vi "Load 16bit Image Stack from Tiff.vi"(0 "path to TIFF file":path=path "/HD1/Users/herbertlooser/Desktop/Ladungsspr焗er.tif", 1 "error in (no error)":errorcluster) -> (5 "I16":i16[][][](array[numeric]), 6 "Directories":cluster{"Tags":T1[]}[](array[cluster]), 7 "error out":errorcluster)   [LabVIEW 2015, in "Tiff reader.lvlib"]
doc: "This .vi is taken from an online tiff reader. It is able to read I16-bit .tiff images."
uses:
  Tiff reader.lvlib
  FieldTypes.ctl
  IFD Entry.ctl
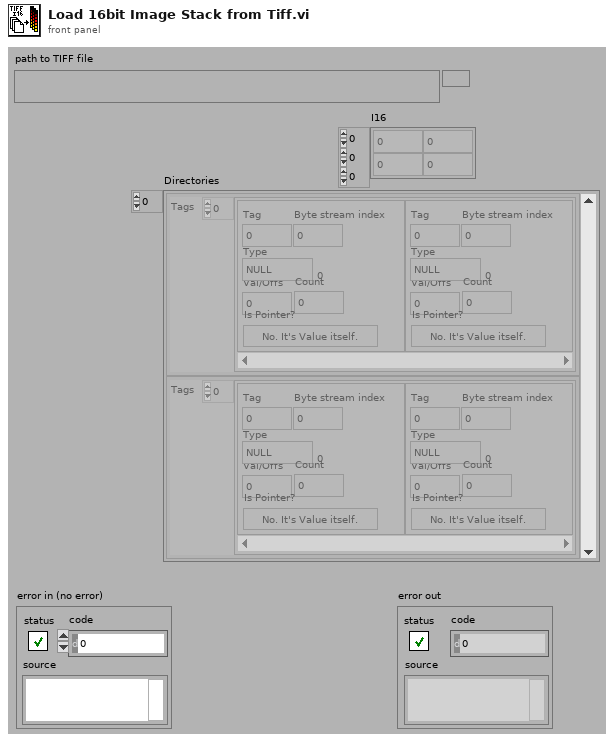
[diagram p1: front panel]
types:
  T1 = typedef "Tiff reader.lvlib/IFD Entry.ctl" = cluster{"Tag":u16, "Type":T2, "Count":u32, "Val/Offs":u32, "Is Pointer?":bool, "Byte stream index":i32}
  T2 = typedef "Tiff reader.lvlib/FieldTypes.ctl" = enum16{"NULL", "U8", "ASCII7", "U16", "U32", "RATIONAL", "SByte(I8)", "Undef(8Bit)", "I16", "I32", "SRat(4B:4B)", "SGL(4Byte)", "DBL(8Byte)"}
  T3 = enum16{"open", "open or create", "create or replace", "create"}
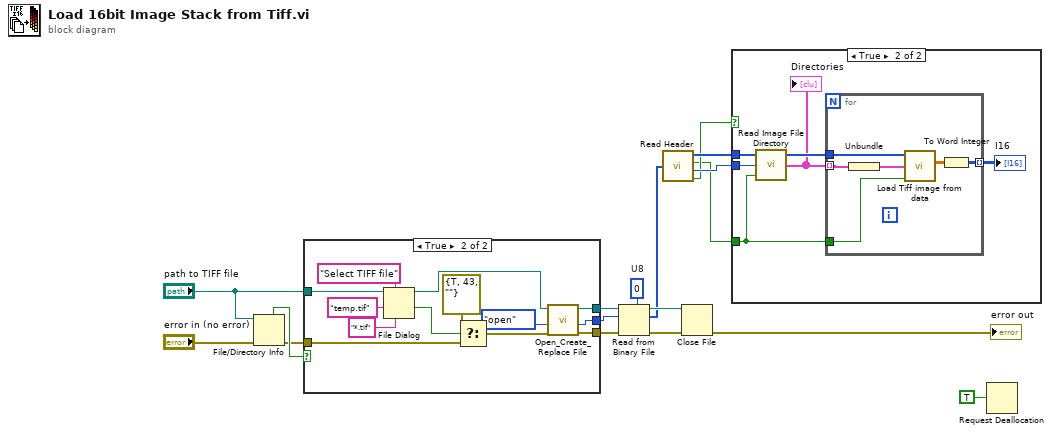
[diagram p0: block diagram]
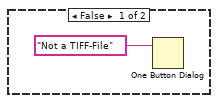
[diagram p2: hidden frame]
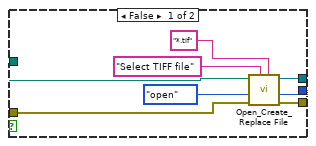
[diagram p3: hidden frame]
diagram:
  w1 = u8 0  # U8
  n1 = File/Directory Info(path="path to TIFF file", error in="error in (no error)") -> (directory=w12:bool, error out=w4:errorcluster)  [unwired: 5 out]
  n2 = case shown="True" w12 {
    tunnel: [w22 w31] -> w17
    tunnel: [w21 w33] -> w16
    tunnel: [w20 w32] -> w13
    tunnel: w4 -> [w19 w29]
    tunnel: "path to TIFF file" -> [w18 w27]
    frame False {
      n3 = call <vilib>:"Open_Create_Replace File.vi"("pattern"="*.tif", "prompt"="Select TIFF file", "error in (no error)"=w19, "function (open:0)"=T3."open", "file path"=w18) -> ("error out"=w20:errorcluster, "file size (bytes)"=w22:i32, "refnum"=w21:refnum<file>)  [unwired: 2 in, 2 out]
    }
    frame True {
      n4 = File Dialog(6:"*.tif" ("pattern"), 7:"Select TIFF file" ("prompt"), 9:"temp.tif" ("default name"), 11:w27) -> (1:w30:bool, 3:w35:path)  [unwired: 1 in, 4 out]
      n5 = Select(t=errorcluster {"status"=TRUE, "code"=43, "source"=""} ("error in (no error)"), s=w30, f=w29) -> (s? t:f=w28:errorcluster)
      n6 = call <vilib>:"Open_Create_Replace File.vi"("error in (no error)"=w28, "function (open:0)"=T3."open", "file path"=w35) -> ("error out"=w32:errorcluster, "file size (bytes)"=w31:i32, "refnum"=w33:refnum<file>)  [unwired: 3 in, 3 out]
    }
  }
  n7 = Read from Binary File(5:w1, 8:w13, 10:w17, 11:w16) -> (0:w14:errorcluster, 2:w2:u8[], 3:w15:refnum<file>)  [unwired: 3 out]
  n8 = call "Read Header.vi"("TIFF Data in"=w2) -> ("TIFF Data out"=w10:u8[], "Litt/BigEnd"=w7:bool, "ImFileDirectOffs"=w9:u32, "IsTIFF?"=w8:bool)
  n9 = Close File(refnum=w15, error in=w14) -> (error out=→"error out":errorcluster)  [unwired: 1 out]
  n10 = case shown="True" w8 {
    tunnel: w10 -> [_ w45]
    tunnel: w9 -> [_ w44]
    tunnel: w7 -> [_ w42]
    frame False {
      n11 = One Button Dialog(message="Not a TIFF-File") -> ()  [unwired: 2 out]
    }
    frame True {
      n12 = call "Read Image File Directory.vi"("Litt/BigEnd"=w42, "Im_File_Dir Offs"=w44, "Image Data in"=w45) -> ("Directories"=w40:cluster{"Tags":T1[]}[], "Image Data out"=w43:u8[])  [unwired: 1 out]
      "Directories" <- w40
      n13 = for {
        tunnel: w43 -> [w51]
        tunnel: w42 -> [w50]
        tunnel: [w48] -> w41 mode=indexing
        tunnel: w40 -> [w47] mode=indexing
        n14 = Unbundle(w47) -> ("Tags"=w46:T1[])
        n15 = call "Load Tiff image from data.vi"("Litt/BigEnd"=w50, "DirEntries"=w46, "Image Data in"=w51) -> ("Gray16/32"=w49:sgl[][])  [unwired: 8 out]
        n16 = To Word Integer(number=w49) -> (16bit integer=w48:i16[][])
      }
      "I16" <- w41
    }
  }
  n17 = Request Deallocation(TRUE ("flag")) -> ()
